vi "Normalize Vector.vi"(8 "error in":errorcluster, 11 "PVector in":refnum<class "PVector.lvclass">) -> (0 "error out":errorcluster, 3 "norm(PVector) out":refnum<class "PVector.lvclass">)   [LabVIEW 2016, in "PVector.lvclass"]
doc: "Set vector V magniture to 1 (change vector <B>V</B> to unit vector <B>u</B>).\nu = V / ||V||"
uses:
  PVector.lvclass
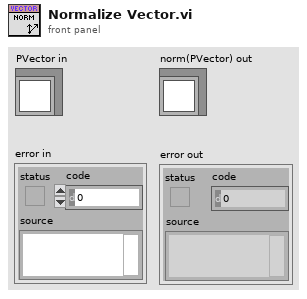
[diagram p1: front panel]
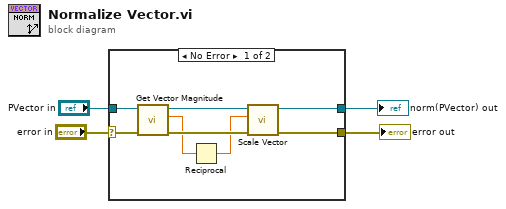
[diagram p0: block diagram]
diagram:
  n1 = case shown="No Error" "error in" {
    selector: "error in" -> [w11 w14]
    tunnel: [w7 w14] -> w3
    tunnel: [w8 w13] -> w1
    tunnel: "PVector in" -> [w12 w13]
    frame No Error {
      n2 = call "Get Vector Magnitude.vi"("error in"=w11, "PVector in"=w12) -> ("error out"=w9:errorcluster, "Mag(V)"=w6:dbl, "PVector out"=w10:refnum<class "PVector.lvclass">)  [unwired: 7 in]
      n3 = Reciprocal(x=w6) -> (1/x=w5:dbl)
      n4 = call "Scale Vector.vi"("error in"=w9, "n (1)"=w5, "PVector V"=w10) -> ("error out"=w7:errorcluster, "PVector nV"=w8:refnum<class "PVector.lvclass">)  [unwired: 7 in]
    }
    frame Error {
    }
  }
  "error out" <- w3
  "norm(PVector) out" <- w1
